vi "CalcTotalScanCount.vi"(0 "Optical Input":T2, 6 "Optical Output":T1, 7 "Total scan count":refnum<vi>, 8 "Number of scans":i32, 10 "x steps":i32, 12 "y steps":i32) -> ()   [LabVIEW 2011]
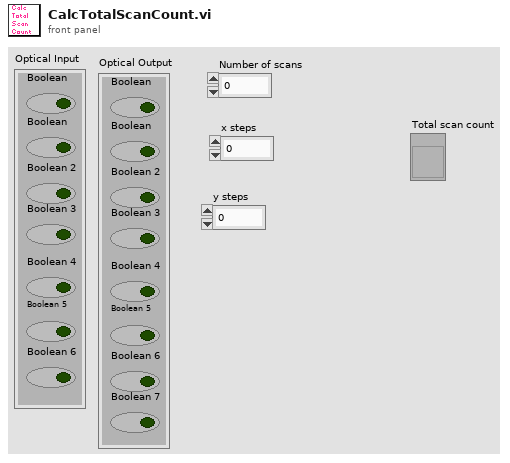
[diagram p1: front panel]
types:
  T1 = cluster{"Boolean":bool, "Boolean":bool, "Boolean 2":bool, "Boolean 3":bool, "Boolean 4":bool, "Boolean 5":bool, "Boolean 6":bool, "Boolean 7":bool}
  T2 = cluster{"Boolean":bool, "Boolean":bool, "Boolean 2":bool, "Boolean 3":bool, "Boolean 4":bool, "Boolean 5":bool, "Boolean 6":bool}
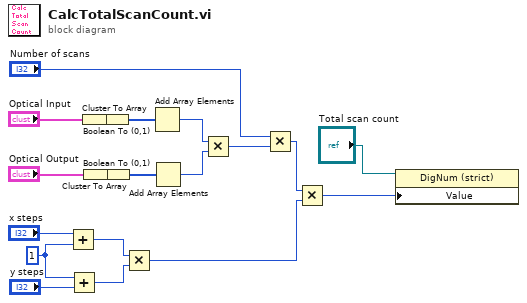
[diagram p0: block diagram]
diagram:
  w6 = 1
  n1 = Add(x="x steps", y=w6) -> (x+y=w5:i32)
  n2 = Add(x=w6, y="y steps") -> (x+y=w4:i32)
  n3 = Cluster To Array(cluster="Optical Input") -> (array=w19:bool[])
  n4 = Cluster To Array(cluster="Optical Output") -> (array=w18:bool[])
  n5 = Boolean To (0,1)(Boolean=w19) -> (0, 1=w17:i16[])
  n6 = Boolean To (0,1)(Boolean=w18) -> (0, 1=w16:i16[])
  n7 = Multiply(x=w5, y=w4) -> (x*y=w2:i32)
  n8 = Add Array Elements(numeric array=w17) -> (sum=w15:i16)
  n9 = Add Array Elements(numeric array=w16) -> (sum=w14:i16)
  n10 = Multiply(x=w15, y=w14) -> (x*y=w9:i16)
  n11 = Multiply(x="Number of scans", y=w9) -> (x*y=w3:i32)
  n12 = Multiply(x=w3, y=w2) -> (x*y=w1:i32)
  n13 = property class="DigNum (strict)"(reference="Total scan count", "Value"=w1) -> ()  [unwired: 1 in, 2 out]
